vi "CANOpen_Get PDO Channel from Name.vi"(11 "PDO Channel Name":string) -> (3 "PDO Channel":i32)   [LabVIEW 2021, in "CANOpen Addon Shared.lvlib"]
uses:
  CANOpen Addon Shared.lvlib
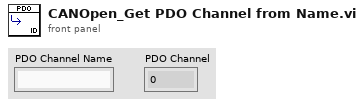
[diagram p1: front panel]
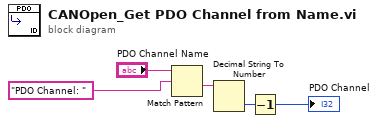
[diagram p0: block diagram]
diagram:
  n1 = Match Pattern(string="PDO Channel Name", regular expression="PDO Channel: ") -> (after substring=w1:string)  [unwired: 1 in, 3 out]
  n2 = Decimal String To Number(string=w1) -> (number=w4:i32)  [unwired: 2 in, 1 out]
  n3 = Decrement(x=w4) -> (x-1=→"PDO Channel":i32)
